vi "Do.vi"(8 "error in (no error)":errorcluster, 10 "Actor in":refnum<class "Actor.lvclass">, 11 "Tiles Info Msg":refnum<class "Tiles Info Msg.lvclass">) -> (0 "error out":errorcluster, 2 "Actor out":refnum<class "Actor.lvclass">)   [LabVIEW 2013, in "Project View.lvlib" / "Tiles Info Msg.lvclass"]
doc: "(<B>Filename</B>: Actor Framework.lvlib:Message.lvclass:Do.vi)\n\nDefines what a message does when it is received by an actor. Generally, a message instructs an actor to invoke one of its methods.\n\nBy default, this method does nothing. A child class must override it to define behavior. Create a child class by using the Actor Framework Message Maker dialog box."
uses:
  Tiles Info Msg.lvclass
  <vilib>/ActorFramework/Actor/Actor.lvclass
  Project View/Project View.lvclass
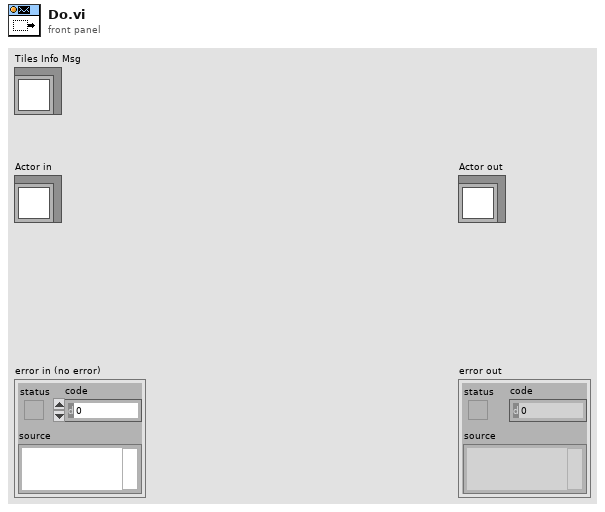
[diagram p1: front panel]
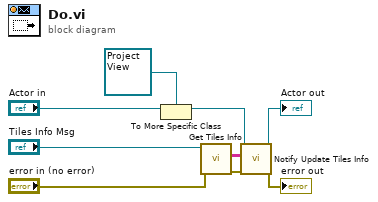
[diagram p0: block diagram]
diagram:
  n1 = To More Specific Class(target class=refnum<class "Project View.lvclass"> refnum ("Project View.lvlib:Project View.lvclass"), reference="Actor in") -> (specific class reference=w7:refnum<class "Project View.lvclass">)  [unwired: 1 in, 1 out]
  n2 = call-dynamic "Get Tiles Info.vi"("error in (no error)"="error in (no error)", "Tiles Info Msg in"="Tiles Info Msg") -> ("error out"=w6:errorcluster, "Tiles Info"=w8:string[][])  [unwired: 7 in, 1 out]
  n3 = call "Notify Update Tiles Info.vi"("error in (no error)"=w6, "Event Data"=w8, "Project View in"=w7) -> ("error out"=→"error out":errorcluster, "Project View out"=→"Actor out":refnum<class "Project View.lvclass">)  [unwired: 7 in]
